vi "Get SMO API Type.vi"(8 "error in (no error)":errorcluster, 11 "Instrument in":refnum<class "Instrument.lvclass">) -> (0 "error out":errorcluster, 2 "API":refnum<class "API.lvclass">, 3 "Instrument out":refnum<class "Instrument.lvclass">)   [LabVIEW 2019, in "Instrument.lvlib" / "Instrument.lvclass"]
doc: "Override this VI to return return the API class used by your instrument."
uses:
  Instrument.lvclass
  Instrument Types/API/API.lvclass
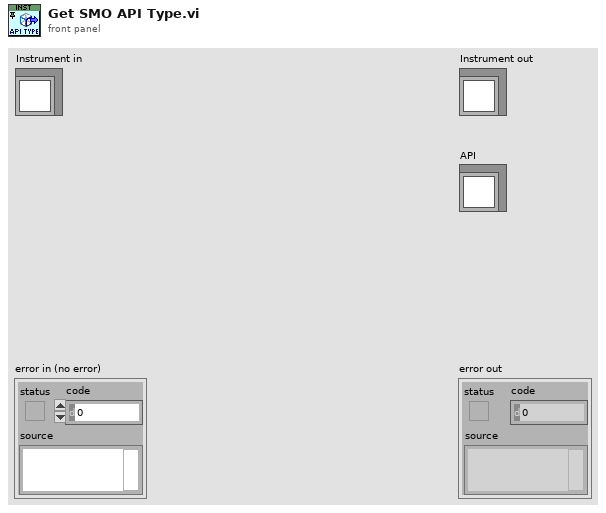
[diagram p1: front panel]
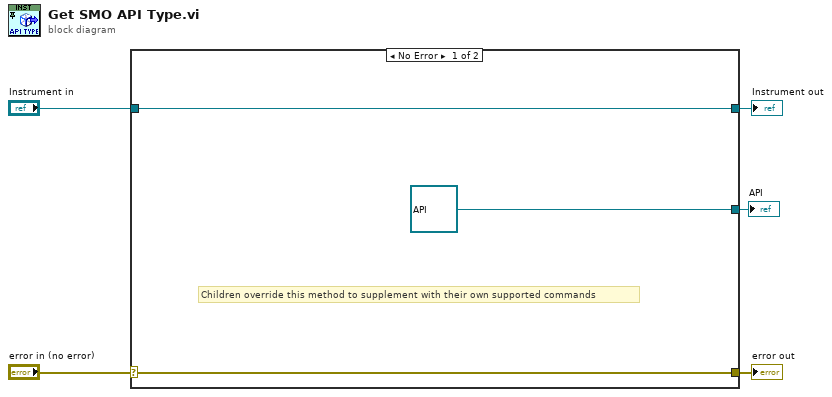
[diagram p0: block diagram]
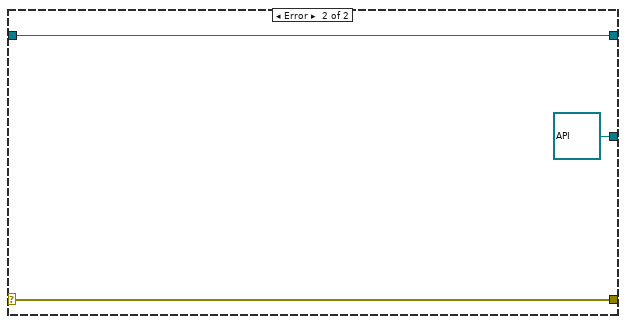
[diagram p2: hidden frame]
diagram:
  n1 = case shown="No Error" "error in (no error)" {
    selector: "error in (no error)" -> [w7 w11]
    tunnel: [w7 w11] -> w4
    tunnel: [w8 w10] -> w2
    tunnel: "Instrument in" -> [w8 w10]
    tunnel: [refnum<class "API.lvclass"> refnum ("API.lvclass") refnum<class "API.lvclass"> refnum ("API.lvclass")] -> w1
    frame No Error {
      # "Children override this method to supplement with their own supported commands"
    }
    frame Error {
    }
  }
  "error out" <- w4
  "Instrument out" <- w2
  "API" <- w1
